vi "generateInformationBox.vi"(9 "Trial Index":i32) -> (0 "Break over":bool, 2 "Information Box":string)   [LabVIEW 2012]
panel:
  in  "Resting":bool
  out "Break start time":u32
  in  "Task description table":string[](array[string])=["Hold still\n\n- Place tip on lower right cross.\n- Hold the tip as still as you can until tone prompt (20 seconds)\n\n", "Mock peel\n\n- Position tip ?? microns over mark.\n- Say \"start\". Wait for start chime.\n- Go down to just above surface, press actuator until tone sounds\n- Lift slowly back up to starting height.\n- Say \"done\".  Wait for chime.\n- Proceed to next mark (repeated 4 times)\n ", "Acquire and Hold Target Point\n\n- Place tip on lower right cross.\n- At tone prompt move clockwise to the next cross \n  and hold as still as you can until the next tone prompt.\n", "Surgery procedure\n\n- Take as long as necessary\n- Say when starting and finishing\n\n\n"]
  # "Locals:"
  # "This table  maps the task codes to text descriptions."
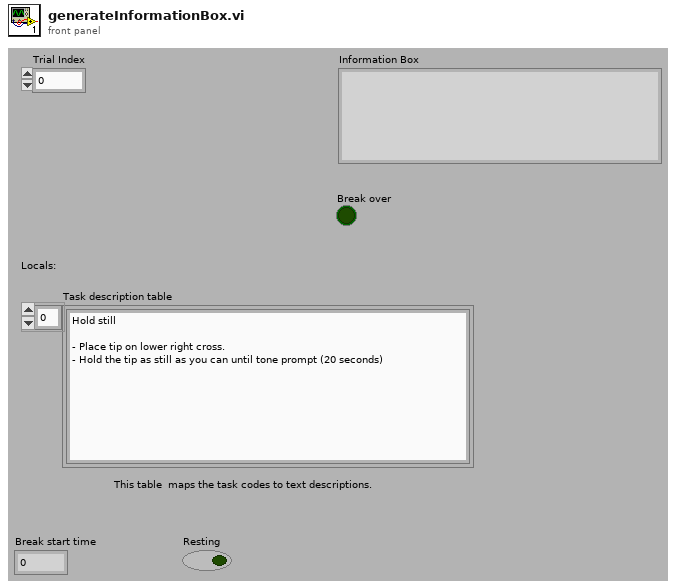
[diagram p1: front panel]
types:
  T1 = typedef "trial_condition.ctl" = cluster{"Type":enum16{"Undefined", "Start", "Normal", "Rest", "Done"}, "Task":u16, "Code":string, "Duration":dbl, "Prompts":u16, "Mode controls":T2, "Variable":bool}
  T2 = typedef "mode_conrols.ctl" = cluster{"Hold":bool, "Cancellation":bool, "Goal filter":bool, "Trigger":bool}
  T3 = enum16{"Undefined", "Start", "Normal", "Rest", "Done"}
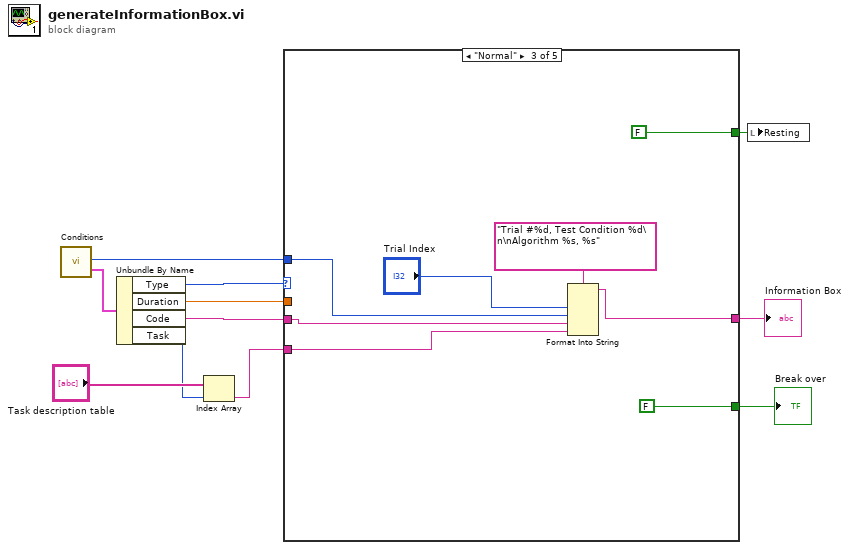
[diagram p0: block diagram]
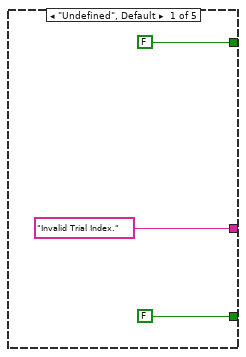
[diagram p2: hidden frame]
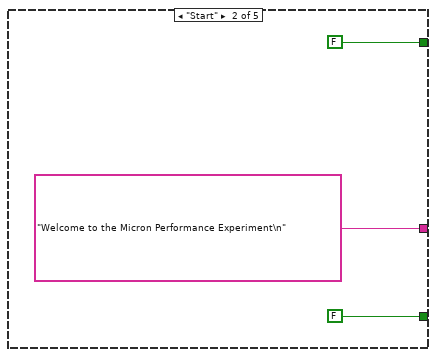
[diagram p3: hidden frame]
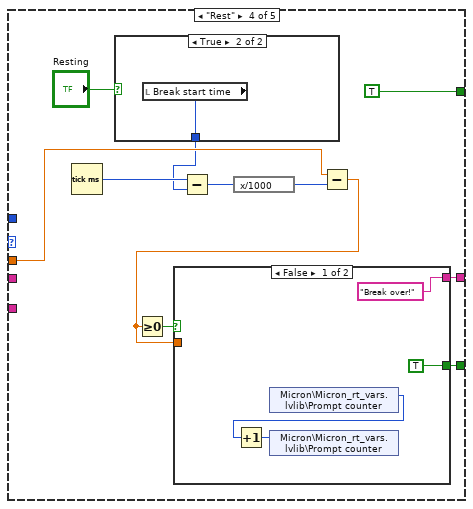
[diagram p4: hidden frame]
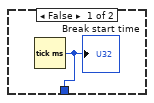
[diagram p5: hidden frame]
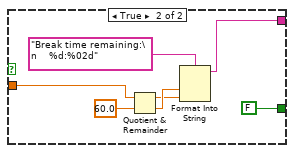
[diagram p6: hidden frame]
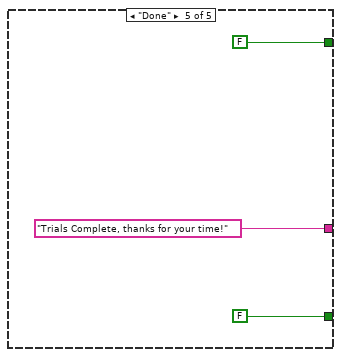
[diagram p7: hidden frame]
diagram:
  n1 = call "Conditions.vi"() -> ("Condition code"=w8:i32, "Current condition"=w7:T1)  [unwired: 2 in, 16 out]
  n2 = Unbundle By Name(w7) -> ("Type"=w6:T3, "Duration"=w3:dbl, "Code"=w4:string, "Task"=w5:u16)
  n3 = Index Array(array="Task description table", index=w5) -> (element=w9:string)
  n4 = case shown="\"Normal\"" w6 {
    tunnel: ["Invalid Trial Index." ("Description") "Welcome to the Micron Performance Experiment\n" ("Description") w22 w35 "Trials Complete, thanks for your time!" ("Description")] -> w10
    tunnel: w9 -> [_ _ w23 _ _]
    tunnel: w8 -> [_ _ w21 _ _]
    tunnel: w4 -> [_ _ w20 _ _]
    tunnel: w3 -> [_ _ _ w34 _]
    tunnel: [FALSE FALSE FALSE TRUE FALSE] -> w2
    tunnel: [FALSE ("Break over") FALSE ("Break over") FALSE ("Break over") w26 FALSE ("Break over")] -> w1
    frame "Undefined", Default {
    }
    frame "Start" {
    }
    frame "Normal" {
      n5 = Format Into String(format string="Trial #%d, Test Condition %d\n\nAlgorithm %s, %s", "Trial Index", w21, w20, w23) -> (resulting string=w22:string)  [unwired: 2 in, 1 out]
    }
    frame "Rest" {
      n6 = Tick Count (ms)() -> (millisecond timer value=w32:u32)
      n7 = case shown="True" "Resting" {
        tunnel: [w37 w38] -> w27
        frame False {
          n8 = Tick Count (ms)() -> (millisecond timer value=w37:u32)
          "Break start time" <- w37
        }
        frame True {
          n9 = local read "Break start time"() -> (w38:u32)
        }
      }
      n10 = Subtract(x=w32, y=w27) -> (x-y=w31:u32)
      n11 = expression code="x/1000"(w31) -> (w30:u32)
      n12 = Subtract(x=w34, y=w30) -> (x-y=w33:dbl)
      n13 = Greater Or Equal To 0?(x=w33) -> (x >= 0?=w36:bool)
      n14 = case shown="False" w36 {
        tunnel: w33 -> [_ w45]
        tunnel: ["Break over!" ("Description") w44] -> w35
        tunnel: [TRUE ("Break over") FALSE ("Break over")] -> w26
        frame False {
          n15 = shared-variable "Micron\\Micron_rt_vars.lvlib\\Prompt counter"() -> (w40:u32)  [unwired: 2 out]
          n16 = Increment(x=w40) -> (x+1=w39:u32)
          n17 = shared-variable "Micron\\Micron_rt_vars.lvlib\\Prompt counter"(w39) -> ()  [unwired: 2 out]
        }
        frame True {
          n18 = Quotient & Remainder(x=w45, y=60.0) -> (x-y*floor(x/y)=w46:dbl, floor(x/y)=w47:dbl)
          n19 = Format Into String(format string="Break time remaining:\n    %d:%02d" ("Description"), w47, w46) -> (resulting string=w44:string)  [unwired: 2 in, 1 out]
        }
      }
    }
    frame "Done" {
    }
  }
  "Information Box" <- w10
  "Break over" <- w1
  n20 = local write "Resting"(w2) -> ()
